vi "Start.vi"(8 "error in":errorcluster, 10 "dt (s)":dbl, 11 "HL Timer in":refnum<class "Loop Timer.lvclass">) -> (0 "error out":errorcluster, 3 "HL Timer out":refnum<class "Loop Timer.lvclass">)   [LabVIEW 2020, in "hse-misc.lvlib" / "Loop Timer.lvclass"]
doc: "Start the timed loop by setting the event timeout to \"0\". The first iteration is executed immediately.\n\n____\nHAMPEL SOFTWARE ENGINEERING v3.8.0 (2023-12-18 14:41)"
uses:
  Loop Timer.lvclass
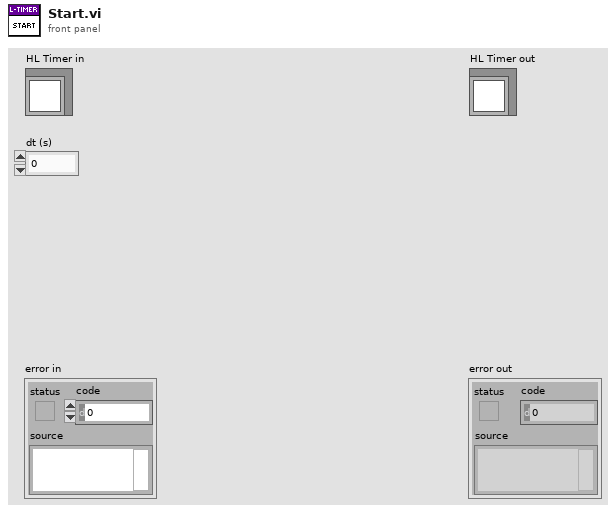
[diagram p1: front panel]
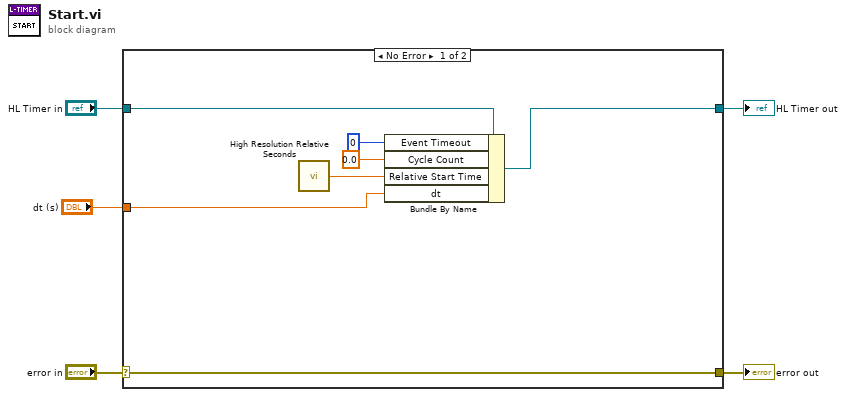
[diagram p0: block diagram]
diagram:
  n1 = case shown="No Error" "error in" {
    selector: "error in" -> [w11 w14]
    tunnel: [w11 w14] -> w4
    tunnel: [w10 w13] -> w2
    tunnel: "HL Timer in" -> [w12 w13]
    tunnel: "dt (s)" -> [w7 _]
    frame No Error {
      n2 = call <vilib>:"High Resolution Relative Seconds.vi"() -> ("relative seconds"=w8:dbl)
      n3 = Bundle By Name(cluster=w12, "Event Timeout"=0, "Cycle Count"=0.0, "Relative Start Time"=w8, "dt"=w7) -> (w10:refnum<class "Loop Timer.lvclass">)
    }
    frame Error {
    }
  }
  "error out" <- w4
  "HL Timer out" <- w2
